vi "Stream Update All Sensors.vi"(8 "error in":errorcluster, 11 "UART port in":T9) -> (0 "error out":errorcluster, 1 "sensors":T1 {"Infrared" format="%02x"}, 3 "UART port out":T9, 5 "Accumulated Distance (mm)":i32, 7 "Accumulated Angle (deg)":i32)   [LabVIEW 2013]
doc: "Reads data from the UART serial port and updates sensors when packets are available.\n\nThis VI assumes that the robot is streaming all sensor data (sensor group 6).\n\nThis VI accumulates distance and angle whenever a new packet is received. While this simplifies most code, which depends on how far the robot has moved, the developer must take account for rollover of signed 32-bit integers if the application has a long running time.\n\nNote that accumulated distance and angle tend to be extremeley inaccurate, since the iRobot looses fractional components of each when it sends a sensor update, and updates are sent at a high rate, resulting in significant roundoff error.\n\nThis VI reads from, but does not write to, the serial port."
uses:
  Advanced/UART/iRobot UART Port Type.ctl
  Sensor Group 6.ctl
  Bumps + Wheel Drops.ctl
  Low-Side Driver + Wheel Overcurrent.ctl
  Buttons.ctl
  Charging State.ctl
  Cargo Bay Digital Inputs.ctl
  Charging Sources Available.ctl
  OI Mode.ctl
  Advanced/UART/iRobot UART Simple Packet Configuration.ctl
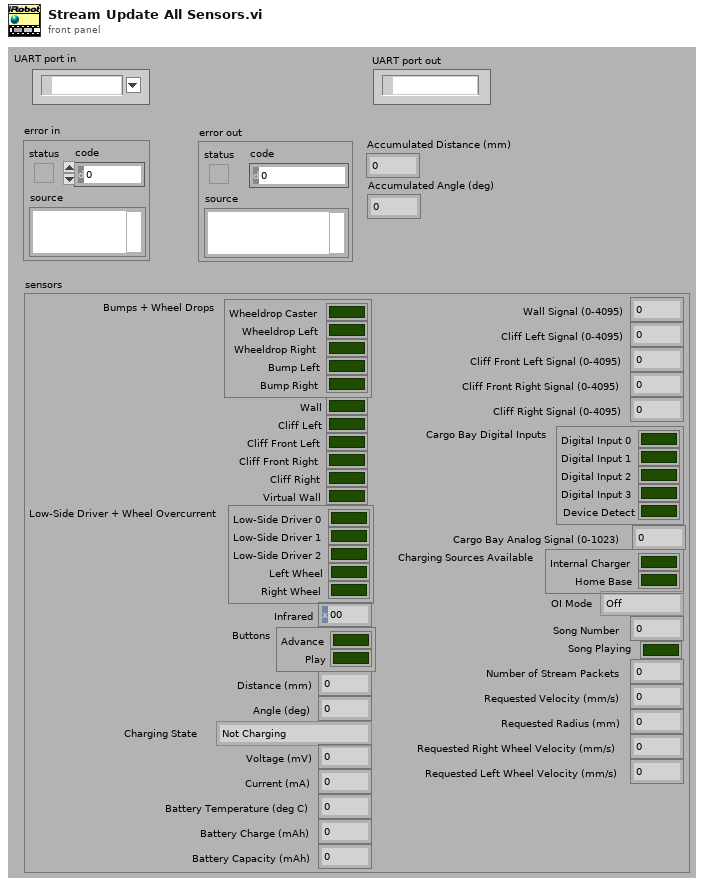
[diagram p1: front panel]
types:
  T1 = typedef "Sensor Group 6.ctl" = cluster{"Bumps + Wheel Drops":T2, "Wall":bool, "Cliff Left":bool, "Cliff Front Left":bool, "Cliff Front Right":bool, "Cliff Right":bool, "Virtual Wall":bool, "Low-Side Driver + Wheel Overcurrent":T3, "Infrared":u8, "Buttons":T4, "Distance (mm)":i32, "Angle (deg)":i32, "Charging State":T5, "Voltage (mV)":u16, "Current (mA)":i16, "Battery Temperature (deg C)":i8, "Battery Charge (mAh)":u16, "Battery Capacity (mAh)":u16, "Wall Signal (0-4095)":u16, "Cliff Left Signal (0-4095)":u16, "Cliff Front Left Signal (0-4095)":u16, "Cliff Front Right Signal (0-4095)":u16, "Cliff Right Signal (0-4095)":u16, "Cargo Bay Digital Inputs":T6, "Cargo Bay Analog Signal (0-1023)":u16, "Charging Sources Available":T7, "OI Mode":T8, "Song Number":u8, "Song Playing":bool, "Number of Stream Packets":u8, "Requested Velocity (mm/s)":i16, "Requested Radius (mm)":i16, "Requested Right Wheel Velocity (mm/s)":i16, "Requested Left Wheel Velocity (mm/s)":i16}
  T2 = typedef "Bumps + Wheel Drops.ctl" = cluster{"Wheeldrop Caster":bool, "Wheeldrop Left":bool, "Wheeldrop Right":bool, "Bump Left":bool, "Bump Right":bool}
  T3 = typedef "Low-Side Driver + Wheel Overcurrent.ctl" = cluster{"Low-Side Driver 0":bool, "Low-Side Driver 1":bool, "Low-Side Driver 2":bool, "Left Wheel":bool, "Right Wheel":bool}
  T4 = typedef "Buttons.ctl" = cluster{"Advance":bool, "Play":bool}
  T5 = typedef "Charging State.ctl" = enum16{"Not Charging", "Reconditioning Charging", "Full Charging", "Trickle Charging", "Waiting", "Charging Fault Condition"}
  T6 = typedef "Cargo Bay Digital Inputs.ctl" = cluster{"Digital Input 0":bool, "Digital Input 1":bool, "Digital Input 2":bool, "Digital Input 3":bool, "Device Detect":bool}
  T7 = typedef "Charging Sources Available.ctl" = cluster{"Internal Charger":bool, "Home Base":bool}
  T8 = typedef "OI Mode.ctl" = enum16{"Off", "Passive", "Safe", "Full"}
  T9 = typedef "iRobot UART Port Type.ctl" = refnum<visa-resource-name>
  T10 = typedef "iRobot UART Simple Packet Configuration.ctl" = cluster{"header":u8[], "create checksum?":bool}
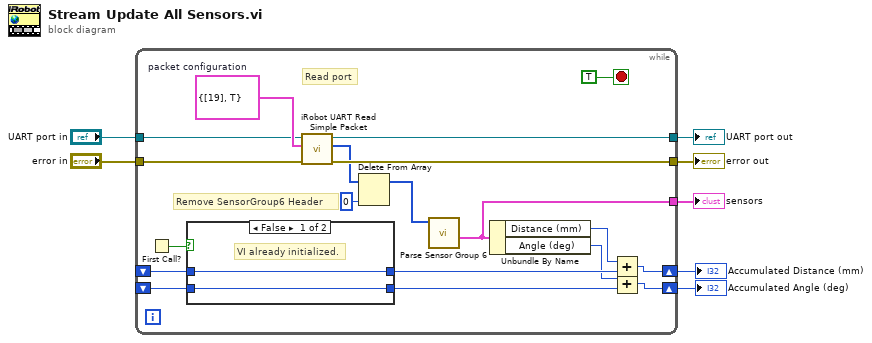
[diagram p0: block diagram]
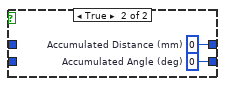
[diagram p2: hidden frame]
diagram:
  n1 = while {
    tunnel: "error in" -> [w13]
    shift-right: [w22] -> w6
    shift-left: _ -> [w20]
    shift-right: [w21] -> w5
    shift-left: _ -> [w19]
    tunnel: [w18] -> w4
    tunnel: [w14] -> w2
    tunnel: "UART port in" -> [w9]
    tunnel: [w8] -> w1
    stop <- TRUE stop-if-true
    w17 = T10 {"header"=[19], "create checksum?"=TRUE}  # packet configuration
    # "Remove SensorGroup6 Header"
    # "Read port"
    n2 = First Call?() -> (First Call?: T/F=w26:bool)
    n3 = case shown="False" w26 {
      tunnel: [w28 w30] -> w24
      tunnel: [w27 w29] -> w23
      tunnel: w20 -> [w28 _]
      tunnel: w19 -> [w27 _]
      frame False {
        # "VI already initialized."
      }
      frame True {
        w29 = 0  # Accumulated Angle (deg)
        w30 = 0  # Accumulated Distance (mm)
      }
    }
    n4 = call "iRobot UART Read Simple Packet.vi"("error in"=w13, "packet configuration"=w17, "UART session"=w9) -> ("error out"=w18:errorcluster, "payload"=w12:u8[], "UART session"=w8:T9)  [unwired: 2 in, 4 out]
    n5 = Delete From Array(array=w12, index=0) -> (array with subset deleted=w10:u8[])  [unwired: 1 in, 1 out]
    n6 = call "Parse Sensor Group 6.vi"("stream in"=w10) -> ("iRobot Sensor Group 6"=w14:T1)  [unwired: 9 in, 1 out]
    n7 = Unbundle By Name(w14) -> ("Distance (mm)"=w16:i32, "Angle (deg)"=w15:i32)
    n8 = Add(x=w16, y=w24) -> (x+y=w22:i32)
    n9 = Add(x=w15, y=w23) -> (x+y=w21:i32)
  }
  "UART port out" <- w1
  "sensors" <- w2
  "error out" <- w4
  "Accumulated Distance (mm)" <- w6
  "Accumulated Angle (deg)" <- w5
